vi "UpdateCPTNested.vi"(8 "error in (no error)":errorcluster, 11 "Caller in":refnum<class "Caller.lvclass">) -> (0 "error out":errorcluster, 3 "Caller out":refnum<class "Caller.lvclass">)   [LabVIEW 2020, in "Caller.lvlib" / "Caller.lvclass"]
uses:
  Caller.lvclass
  C:/Program Files/National Instruments/LabVIEW 2020/vi.lib/ActorFramework/Actor/Actor.lvclass
  Caller.lvclass/Caller.ctl
  <vilib>/ActorFramework/Actor/Actor.lvclass
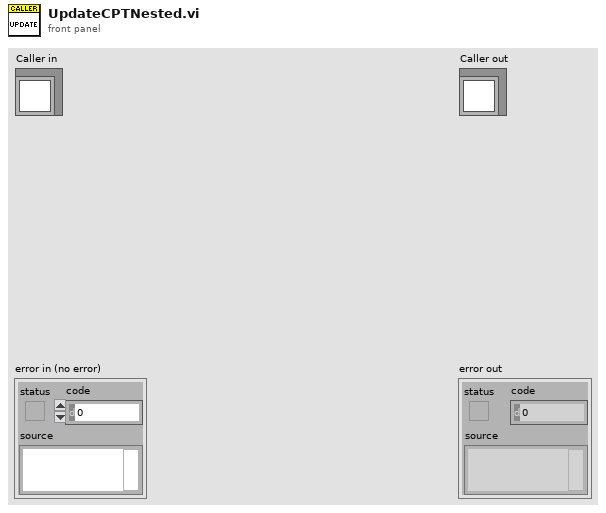
[diagram p1: front panel]
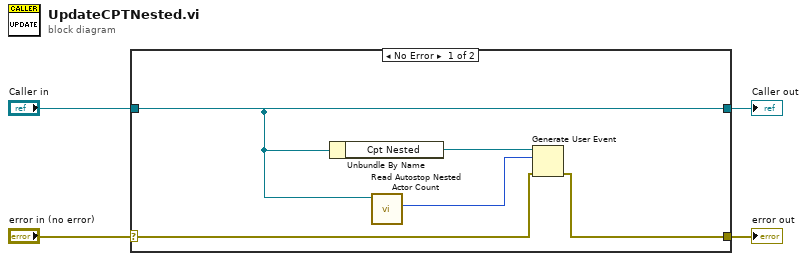
[diagram p0: block diagram]
diagram:
  n1 = case shown="No Error" "error in (no error)" {
    selector: "error in (no error)" -> [w6 w11]
    tunnel: [w5 w11] -> w3
    tunnel: [w9 w10] -> w1
    tunnel: "Caller in" -> [w9 w10]
    frame No Error {
      n2 = Unbundle By Name(w9) -> ("Cpt Nested"=w8:refnum<user-event>)
      n3 = call <vilib>:"Read Autostop Nested Actor Count.vi"("Actor in"=w9) -> ("Count"=w7:i32)  [unwired: 10 in]
      n4 = Generate User Event(user event=w8, event data cluster=w7, error in=w6) -> (error out=w5:errorcluster)  [unwired: 1 in, 1 out]
    }
    frame Error {
    }
  }
  "error out" <- w3
  "Caller out" <- w1
